vi "QuinticHermiteSpline_makeHermiteBasis.vi"() -> (3 "HermiteBasis":T1)   [LabVIEW 2019, in "Trajectory_Library.lvlib"]
doc: "Returns the hermite basis matrix for quintic hermite spline interpolation.\n\nParameters:\n - none -\n\nReturns:\n - HermiteBasis - The hermite basis matrix for quintic hermite spline interpolation."
uses:
  Trajectory_Library.lvlib
  <vilib>/Analysis/Matrix/Datatypes/RealMatrix.ctl
  <vilib>/Analysis/Matrix/NI_Matrix.lvlib
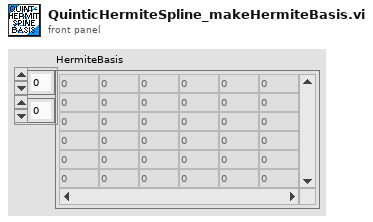
[diagram p1: front panel]
types:
  T1 = typedef "NI_Matrix.lvlib/RealMatrix.ctl" = dbl[][]
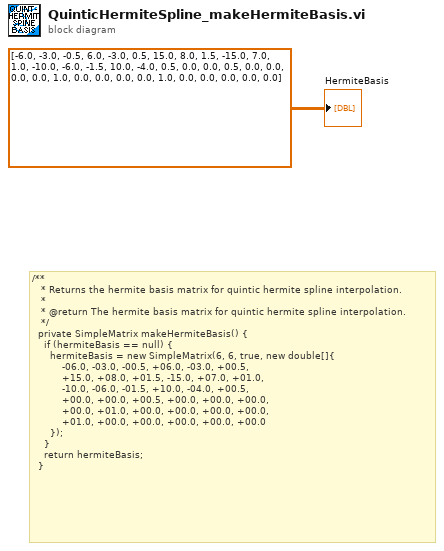
[diagram p0: block diagram]
diagram:
  # "/**\n   * Returns the hermite basis matrix for quintic hermite spline interpolation.\n   *\n   * @return The hermite basis matrix for quintic hermite spline interpolation.\n   */\n  private SimpleMatrix makeHermiteBasis() {\n    if (hermiteBasis == null) {\n      hermiteBasis = new SimpleMatrix(6, 6, true, new double[]{\n          -06.0, -03.0, -00.5, +06.0, -03.0, +00.5,\n          +15.0, +08.0, +01.5, -15.0, +07.0, +01.0,\n          -10.0, -06.0, -01.5, +10.0, -04.0, +00.5,\n          +00.0, +00.0, +00.5, +00.0, +00.0, +00.0,\n          +00.0, +01.0, +00.0, +00.0, +00.0, +00.0,\n          +01.0, +00.0, +00.0, +00.0, +00.0, +00.0\n      });\n    }\n    return hermiteBasis;\n  }"
  "HermiteBasis" <- T1 [[-6.0, -3.0, -0.5, 6.0, -3.0, 0.5], [15.0, 8.0, 1.5, -15.0, 7.0, 1.0], [-10.0, -6.0, -1.5, 10.0, -4.0, 0.5], [0.0, 0.0, 0.5, 0.0, 0.0, 0.0], [0.0, 1.0, 0.0, 0.0, 0.0, 0.0], [1.0, 0.0, 0.0, 0.0, 0.0, 0.0]] ("HermiteBasis")
